vi "DS345.set ramp.vi"(0 "i ref in":refnum<vi>, 2 "sampleFrequency [Hz]":dbl=1000000.0 format="%.2f", 4 "delay [us]":dbl=1.0 format="%.2f", 5 "error in (no error)":errorcluster, 6 "x1 [us]":dbl=1.0 format="%.2f", 7 "x2 [us]":dbl=1.0 format="%.2f", 8 "y1 [V]":dbl=1.0 format="%.2f", 9 "y2 [V]":dbl=1.0 format="%.2f") -> (14 "i ref out":refnum<vi>, 19 "error out":errorcluster)   [LabVIEW 2014, in "DS345.lvlib"]
doc: "Switches the DS345 into delay gate generator mode and sets a ramp waveform for output. The DS345 outputs the ramp waveform when it is externally triggered. \n\nThe ramp waveform is the following:\nt=0us; U=0V\nt=delay; U=0V\nt=delay+x1; U=y1;\nt=delay+x2; U=y1;\nt=delay+x2+1000000us/(sample frequency); U=0V;\n\nNote, that the sample frequency is important. It determines the granularity of the time resolution. However, the values for (delay+x1+x2)/(sample frequency) must be smaller than 16296."
uses:
  DS345.lvlib
  CSCore/CSSystem/CoreLib/CoreLib.lvlib
  CSCore/CSSystem/CoreDefs/CoreDefs.error_type.ctl
  CSCore/CSApplicationBaseClasses/AFGBase/AFGBase.lvlib
  CSCore/CSApplicationBaseClasses/AFGBase/AFGBase.waveformType.ctl
  CSCore/CSApplicationBaseClasses/DeviceBase/DeviceBase.lvlib
  CSlibraries/UtilityLib/UtilityLib.valueStatus.ctl
  CSlibraries/UtilityLib/UtilityLib.lvlib
  CSCore/CSApplicationBaseClasses/DeviceBase/DeviceBase.deviceState.ctl
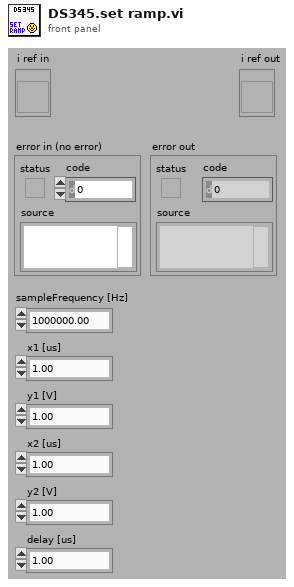
[diagram p1: front panel]
types:
  T1 = typedef "AFGBase.lvlib/AFGBase.waveformType.ctl" = enum16{"sine", "square", "ramp", "pulse", "noise", "DC", "arbitrary", "triangle", "ramp_up", "ramp_down", "amplitude modulation"}
  T2 = typedef "UtilityLib.lvlib/UtilityLib.valueStatus.ctl" = enum16{"no info available", "stand by/off", "on", "warning", "alarm/malfunction", "not implemented", "user action required", "important information", "system default", "control default", "indicator default", "button default"}
  T3 = typedef "CoreDefs.error_type.ctl" = enum16{"no error", "can't load process", "can't unload process", "process does not exist", "can't install process", "can't remove process", "unknown function", "time out", "can't execute function", "duplicate queue name", "super not found", "caller queue invalid", "can't ping process", "unknown error", "VISA Error", "VISA timeout", "GPIB timeout", "GPIB error", "communication error", "data type mismatch", "can't read data from OPC server", "can't write data to OPC server", "OET error", "function not implemented", "process already exists", "invalid Shared Variable name", "error writing Shared Variable", "error reading Shared Variable", "invalid client name", "corrupt database", "unknown class", "call not authorized", "parameter out of range", "OET timeout: can't get data to modify", "invalid queue name", "requested operation incompatible with current state", "event undefined", "event disabled", "state undefined", "caller is not a friend", "EventBuilder: bad eventID", "EventBuilder: no DAQ devices", "a thread must not stop itself", "UNUSED ELEMENT4", "DiscArchiver: eventData incomplete", "DiscArchiver: eventData does not belong to run", "DiscArchiver: can't open file", "DiscArchiver: can't write to file", "DiscArchiver: available disc space low", "can't acquire semaphore", "error reading data from database", "notifier object is not existing", "can't register process", "can't unregister process", "illegal event type", "object disabled", "object already exists", "can't change state", "Instrument not found", "no connection to remote node", "invalid reference", "N/A", "UNUSED ELEMENT 1", "element not found", "illegal TCP/IP connection detected", "object does not exist", "invalid access ID", "unknown CS system", "invalid privilige", "unsupported data type", "unsupported server type", "IO server already exists", "Shared Variable already exists"}
  T4 = typedef "DeviceBase.lvlib/DeviceBase.deviceState.ctl" = i16
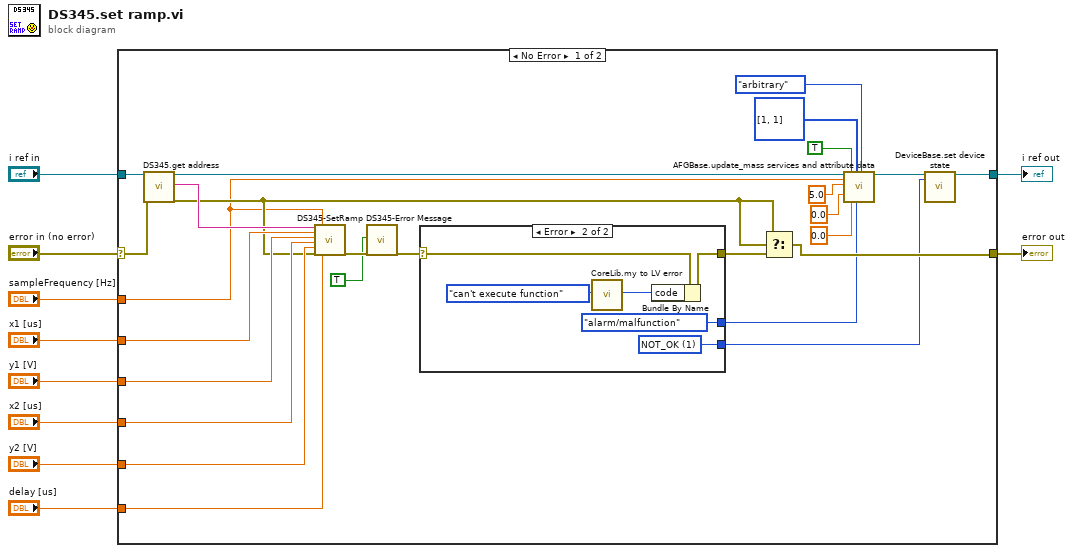
[diagram p0: block diagram]
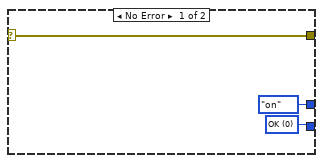
[diagram p2: hidden frame]
diagram:
  n1 = case shown="No Error" "error in (no error)" {
    selector: "error in (no error)" -> [w23 w46]
    tunnel: [w36 w46] -> w10
    tunnel: "i ref in" -> [w34 w47]
    tunnel: "x1 [us]" -> [w33 _]
    tunnel: "y1 [V]" -> [w32 _]
    tunnel: "x2 [us]" -> [w31 _]
    tunnel: "y2 [V]" -> [w30 _]
    tunnel: "sampleFrequency [Hz]" -> [w14 _]
    tunnel: "delay [us]" -> [w28 _]
    tunnel: [w11 w47] -> w2
    frame No Error {
      n2 = call "DS345.get address.vi"("i ref in"=w34, "error in (no error)"=w23) -> ("i ref out"=w16:refnum<vi>, "address"=w35:string, "error out"=w29:errorcluster)  [unwired: 15 in]
      n3 = call "DS345-SetRamp.vi"("address string"=w35, "x1 [us]"=w33, "y1 [V]"=w32, "x2 [us]"=w31, "y2 [V]"=w30, "error in (no error)"=w29, "sampleFrequency [Hz]"=w14, "delay [us]"=w28) -> ("error out"=w27:errorcluster)  [unwired: 10 in, 1 out]
      n4 = call "DS345-Error Message.vi"("addMessageToSource"=TRUE ("add message to source"), "error in (no error)"=w27) -> ("error out"=w26:errorcluster)  [unwired: 14 in, 3 out]
      n5 = case shown="Error" w26 {
        selector: w26 -> [w39 w45]
        tunnel: [w39 w44] -> w24
        tunnel: [UtilityLib.valueStatus."on" ("valueStatus") UtilityLib.valueStatus."alarm/malfunction" ("valueStatus")] -> w13
        tunnel: [w37 w40] -> w12
        frame No Error {
          w37 = T4 0 items=["ERROR"=-1, "OK"=0, "NOT_OK"=1] ("deviceState")
        }
        frame Error {
          w40 = T4 1 items=["ERROR"=-1, "OK"=0, "NOT_OK"=1] ("deviceState")
          n6 = call "CoreLib.my to LV error.vi"("ErrorTypes"=CoreDefs.error_type."can't execute function") -> ("LV error code"=w43:i32)  [unwired: 17 in, 1 out]
          n7 = Bundle By Name(cluster=w45, "code"=w43) -> (w44:errorcluster)
        }
      }
      n8 = Select(t=w29, s=w29, f=w24) -> (s? t:f=w36:errorcluster)
      n9 = call "AFGBase.update_mass services and attribute data.vi"("i ref in"=w16, "frequency"=w14, "amplitude"=5.0, "phase"=0.0, "enableOutput"=TRUE, "DCOffset"=0.0, "trigger"=i16[] [1, 1], "valueStatus"=w13, "waveformType"=AFGBase.waveformType."arbitrary") -> ("i ref out"=w17:refnum<vi>)  [unwired: 8 in, 2 out]
      n10 = call "DeviceBase.set device state.vi"("i ref in"=w17, "deviceState"=w12) -> ("i ref out"=w11:refnum<vi>)  [unwired: 15 in, 2 out]
    }
    frame Error {
    }
  }
  "error out" <- w10
  "i ref out" <- w2
